vi "Test Count Progress on zero Tests.vi"(8 "error in (no error)":errorcluster, 11 "Result Model Tests in":refnum<class "Result Model Statistics.lvclass">) -> (0 "error out":errorcluster, 3 "Result Model Tests out":refnum<class "Result Model Statistics.lvclass">)   [LabVIEW 2020, in "Result Model Statistics.lvclass"]
uses:
  Result Model Statistics.lvclass
  C:/Program Files (x86)/National Instruments/LabVIEW 2020/vi.lib/Astemes/LUnit/Test Case.lvclass
  Result Model/Result Model.lvclass
  <vilib>/Astemes/LUnit/Test Case.lvclass/Test Case.ctl
  206db1ee-aa99-40b9-8881-171f2a77c34b.vi
  <vilib>/Astemes/LUnit/Palette/Pass.vi
  <vilib>/Astemes/LUnit/Palette/Fail.vi
  <vilib>/Astemes/LUnit/Compare Variants.vi
  <vilib>/Astemes/LUnit/Describe Comparison.vi
  <vilib>/Astemes/LUnit/Set Assertion Type.vi
  <vilib>/Astemes/LUnit/Add test result.vi
  <vilib>/Astemes/LUnit/Variant to string.vi
  <vilib>/Astemes/LUnit/LUnit Record Assertion Result.vi
  <vilib>/Astemes/LUnit/LUnit Aggregate Assertion Results.vi
  <vilib>/Astemes/LUnit/Method Result/LUnit Merge Status.vi
  <vilib>/Astemes/LUnit/LUnit Concatenate result strings.vi
  <vilib>/Utility/Data Type/Get Type Information.vi
  <vilib>/Utility/LVClass/Get LV Class Name.vi
  Result Model Statistics.lvclass/Result Model Statistics.ctl
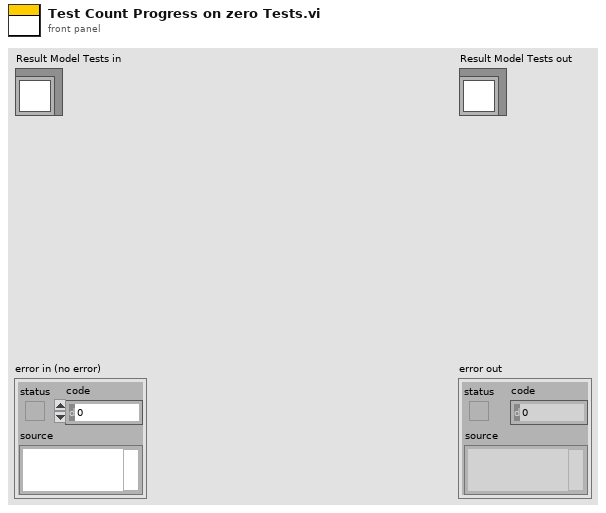
[diagram p1: front panel]
types:
  T1 = typedef "Result Model.lvclass/Statistics.ctl" = cluster{"Method Count":u32, "Executed Methods":u32, "Passed Methods":u32, "Failed Methods":u32, "Method Errors":u32, "Skipped Method":u32, "Progress [%]":dbl}
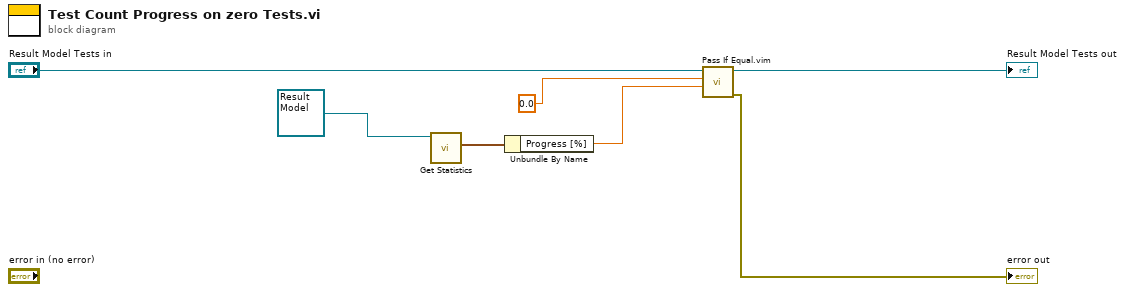
[diagram p0: block diagram]
diagram:
  n1 = call "Get Statistics.vi"("Result Model in"=refnum<class "Result Model.lvclass"> refnum) -> ("Results"=w4:T1)  [unwired: 10 in]
  n2 = Unbundle By Name(w4) -> ("Progress [%]"=w3:dbl)
  n3 = call "Pass If Equal.vim"("Actual"=w3, "Expected"=0.0 ("Method Count"), "LUnit Test Case In"="Result Model Tests in") -> ("error out"=→"error out":errorcluster, "LUnit Test Case Out"=→"Result Model Tests out":refnum<class "Result Model Statistics.lvclass">)  [unwired: 7 in]
